vi "PowerMeterInit.vi"(1 "错误输入（无错误）":errorcluster) -> (0 "错误输出":errorcluster)   [LabVIEW 2018]
panel:
  out "数据输入":string
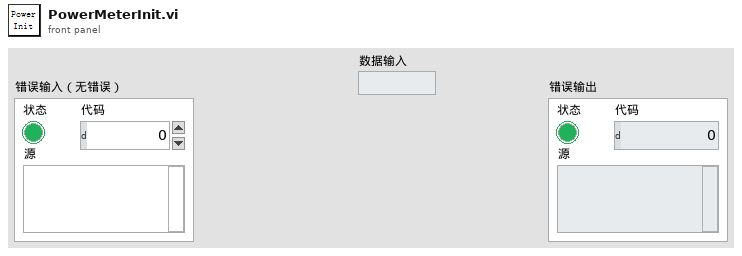
[diagram p1: front panel]
types:
  T1 = enum16{"Standard", "Buffered", "CRLF", "Immediate"}
  T2 = typedef "IMAQ Image.ctl" = refnum<image>
  T3 = cluster{"示波器":cluster{"Channel (0:Channel 1)":enum16{"Channel 1", "Channel 2", "Channel 3", "Channel 4"}, "电压范围":dbl, "触发电压":dbl, "时间范围":dbl, " 示波器VISA":refnum<visa-resource-name>, "电压范围 标签":u64, "时间范围 标签":u64}, "光谱仪":cluster{"Channel (0:Channel 1)":enum16{"Channel 1", "Channel 2", "Channel 3", "Channel 4"}, "电压范围":u64, "触发电压":u64, "时间范围":u64}, " 近场相机":cluster{"曝光时间":i32, "模拟增益":i32, "控制套接字":i32, "IP 地址":string, " 采集套接字":i32, "  版本号":i32, "ImageData":T2, "  增益最大":i32, "  增益最小":i32, " 曝光最大":i32, " 曝光最小":i32, " 帧速":i32, " 同步切换":i32, "  曝光缩放":i32}, " 偏振仪":cluster{"电压范围":u64, "触发电压":u64, "时间范围":u64, "波长范围":enum16{"可见光 400-700nm", "近红外 700-1100nm"}}, " 功率计":cluster{"通道":enum16{"Channel 1", "Channel 2"}, "工作波长":u32, "单位":u64, "时间范围":u64, "IP地址":string, "端口":u32}, "能量计":cluster{"通道":enum16{"Channel 1", "Channel 2"}, "工作波长":u32, "单位":u64, "时间范围":u64, "IP地址":string, "端口":u32, "能量计量程":enum16{"200uJ", "20uJ", "2uJ", "200nJ"}}, "电机":cluster{"Channel (0:Channel 1)":enum16{"Channel 1", "Channel 2", "Channel 3", "Channel 4"}, "电压范围":u64, "触发电压":u64, "时间范围":u64}, " 远场相机":cluster{"曝光时间":i32, "模拟增益":i32, "控制套接字":i32, "IP 地址":string, " 采集套接字":i32, "  版本号":i32, "ImageData":T2, "  增益最大":i32, "  增益最小":i32, " 曝光最大":i32, " 曝光最小":i32, " 帧速":i32, " 同步切换":i32, "  曝光缩放":i32}}
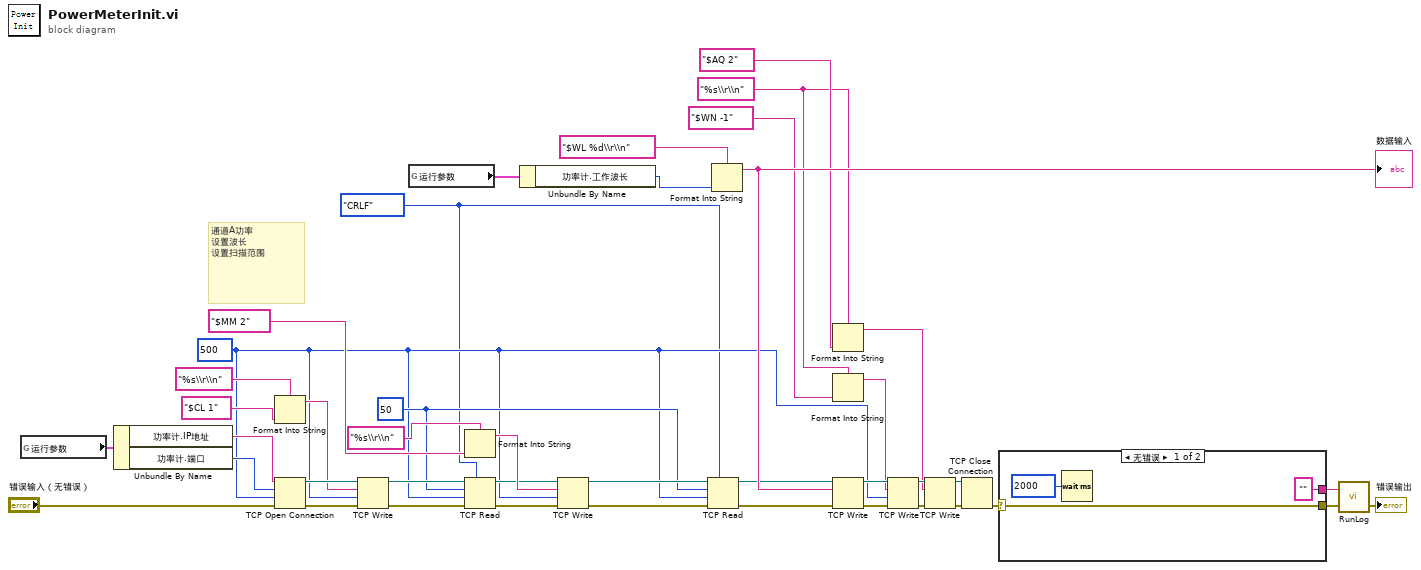
[diagram p0: block diagram]
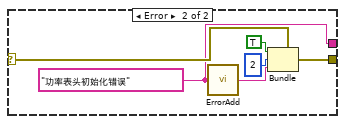
[diagram p2: hidden frame]
diagram:
  w3 = 50 ("读取的字节")
  w1 = T1."CRLF" ("模式（标准）")
  w13 = "%s\\r\\n" ("格式字符串")
  w2 = 500
  # "通道A功率\n设置波长\n设置扫描范围"
  n1 = global read "参数.vi" "运行参数"() -> (w23:T3)
  n2 = Unbundle By Name(w23) -> ("功率计.IP地址"=w22:string, "功率计.端口"=w17:u32)
  n3 = Format Into String(format string="%s\\r\\n" ("格式字符串"), "$CL 1" ("输入 1")) -> (resulting string=w38:string)  [unwired: 2 in, 1 out]
  n4 = TCP Open Connection(address=w22, remote port or service name=w17, timeout ms (60000)=w2, error in (no error)="错误输入（无错误）") -> (connection ID=w39:refnum<k5>, error out=w37:errorcluster)  [unwired: 1 in]
  n5 = TCP Write(connection ID=w39, data in=w38, error in (no error)=w37, 9:w2) -> (connection ID out=w11:refnum<k5>, error out=w9:errorcluster)  [unwired: 1 out]
  n6 = global read "参数.vi" "运行参数"() -> (w32:T3)
  n7 = Format Into String(format string="%s\\r\\n" ("格式字符串"), "$MM 2" ("输入 1")) -> (resulting string=w41:string)  [unwired: 2 in, 1 out]
  n8 = TCP Read(connection ID=w11, bytes to read=w3, error in (no error)=w9, 7:w1, 9:w2) -> (connection ID out=w10:refnum<k5>, error out=w8:errorcluster)  [unwired: 1 out]
  n9 = Unbundle By Name(w32) -> ("功率计.工作波长"=w27:u32)
  n10 = TCP Write(connection ID=w10, data in=w41, error in (no error)=w8, 9:w2) -> (connection ID out=w7:refnum<k5>, error out=w4:errorcluster)  [unwired: 1 out]
  n11 = TCP Read(connection ID=w7, bytes to read=w3, error in (no error)=w4, 7:w1, 9:w2) -> (connection ID out=w6:refnum<k5>, error out=w5:errorcluster)  [unwired: 1 out]
  n12 = Format Into String(format string="$WL %d\\r\\n" ("格式字符串"), w27) -> (resulting string=w26:string)  [unwired: 2 in, 1 out]
  "数据输入" <- w26
  n13 = Format Into String(format string=w13, "$AQ 2" ("数据输入")) -> (resulting string=w12:string)  [unwired: 2 in, 1 out]
  n14 = Format Into String(format string=w13, "$WN -1" ("数据输入")) -> (resulting string=w15:string)  [unwired: 2 in, 1 out]
  n15 = TCP Write(connection ID=w6, data in=w26, error in (no error)=w5) -> (connection ID out=w25:refnum<k5>, error out=w24:errorcluster)  [unwired: 1 in, 1 out]
  n16 = TCP Write(connection ID=w25, data in=w15, error in (no error)=w24, 9:w2) -> (connection ID out=w21:refnum<k5>, error out=w20:errorcluster)  [unwired: 1 out]
  n17 = TCP Write(connection ID=w21, data in=w12, error in (no error)=w20) -> (connection ID out=w19:refnum<k5>, error out=w18:errorcluster)  [unwired: 1 in, 1 out]
  n18 = TCP Close Connection(connection ID=w19, error in (no error)=w18) -> (error out=w31:errorcluster)  [unwired: 1 in, 1 out]
  n19 = case shown="无错误" w31 {
    selector: w31 -> [w45 w48]
    tunnel: [w45 w47] -> w29
    tunnel: ["" ("source") w46] -> w30
    frame No Error {
      n20 = Wait (ms)(milliseconds to wait=u32 2000 ("等待时间（毫秒）")) -> ()  [unwired: 1 out]
    }
    frame Error {
      w46 = "功率表头初始化错误" ("source")
      n21 = call "ErrorAdd.vi"("source"=w46) -> ("Errorout Souce"=w49:string)
      n22 = Bundle(cluster=w48, "status"=TRUE, "code"=2, "source"=w49) -> (w47:errorcluster)
    }
  }
  n23 = call "RunLog.vi"("error in"=w29, "Message"=w30) -> ("error out"=→"错误输出":errorcluster)  [unwired: 1 in]
